vi "MeasurementLink Common Proto Generator.vi"(0 "Proto File Path":path[](array[path]), 1 "Generated Library Full Name":string, 3 "Generate":enum16{"gRPC Server", "gRPC Client", "Both"}(ring), 5 "Import Paths":path[](array[path]), 7 "Prototype Library":path, 9 "Target Project":path, 11 "error in (no error)":errorcluster) -> (15 "error out":errorcluster)   [LabVIEW 2020]
uses:
  <vilib>/regexp/Match Regular Expression.xnode
panel:
  in  "Debug - Prompt before deleting disk content? (F)":bool
  in  "Debug - Leave Project Open? (F)":bool
  # "Ignored for servers as of v0.5.2.2"
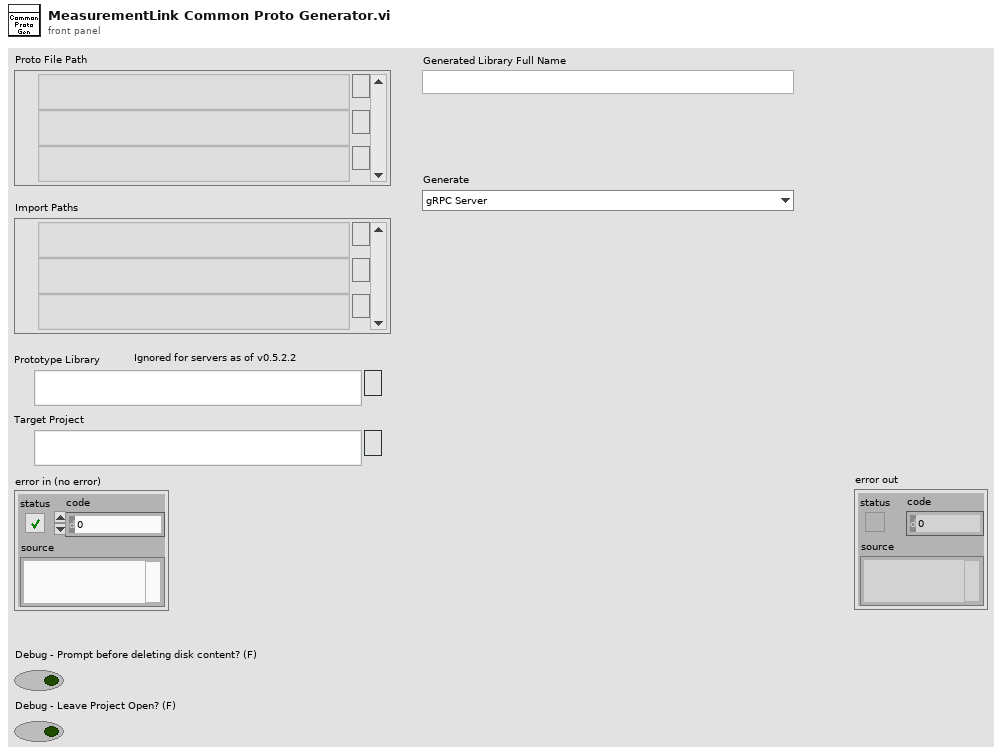
[diagram p1: front panel]
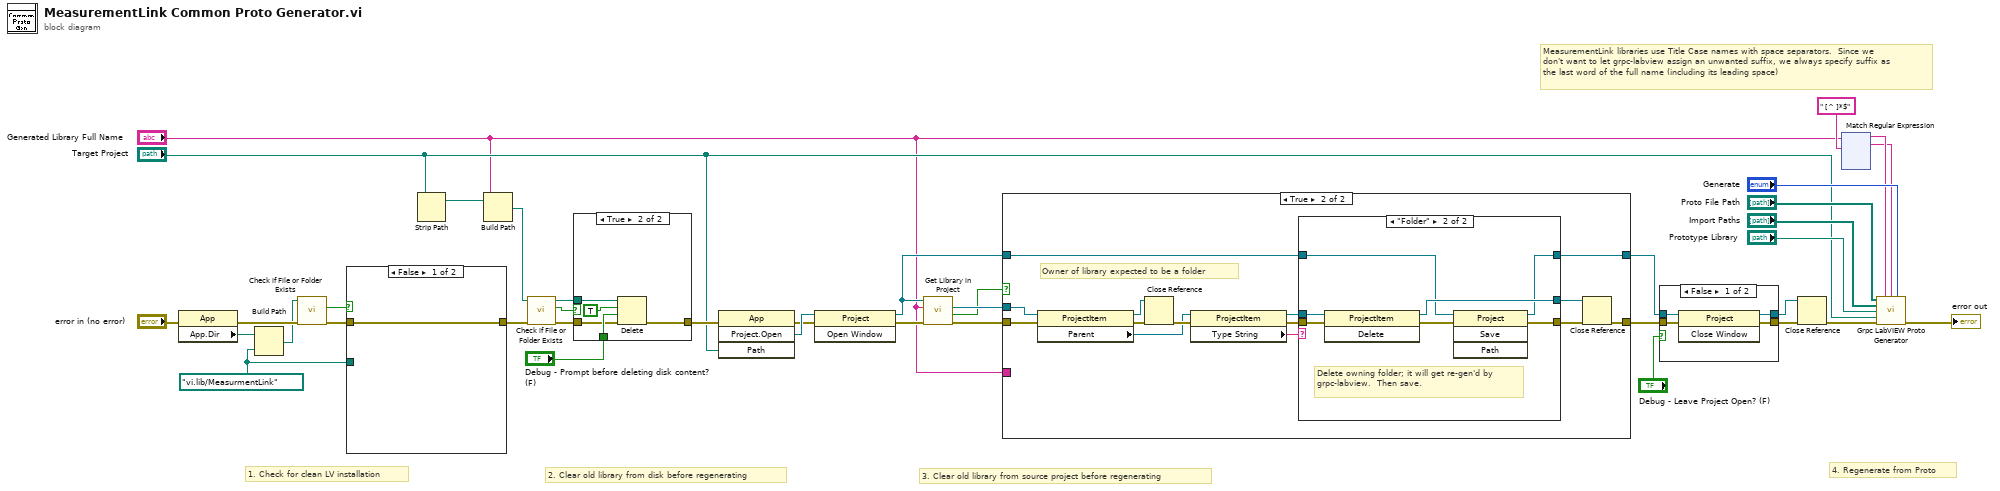
[diagram p0: block diagram]
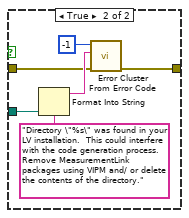
[diagram p2: hidden frame]
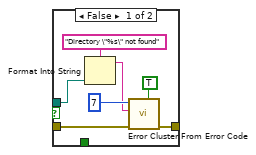
[diagram p3: hidden frame]
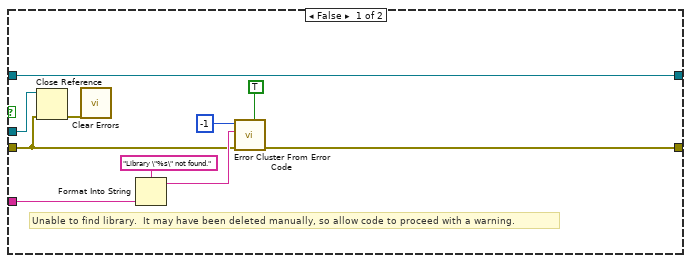
[diagram p4: hidden frame]
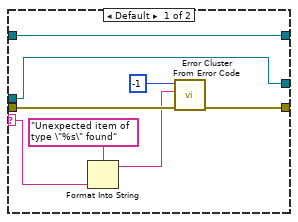
[diagram p5: hidden frame]
diagram:
  w6 = path "vi.lib/MeasurmentLink" ("Target Project")
  # "MeasurementLink libraries use Title Case names with space separators.  Since we don't want to let grpc-labview assign an unwanted suffix, we always specify suffix as the last word of the full name (including its leading space)"
  # "4. Regenerate from Proto"
  # "3. Clear old library from source project before regenerating"
  # "2. Clear old library from disk before regenerating"
  # "1. Check for clean LV installation"
  n1 = property class="App"(error in="error in (no error)") -> (error out=w11:errorcluster, "App.Dir"=w13:path)  [unwired: 1 in, 1 out]
  n2 = Build Path(base path=w13, name or relative path=w6) -> (appended path=w10:path)
  n3 = call <vilib>:"Check if File or Folder Exists.vi"("error in (no error)"=w11, "path"=w10) -> ("error out"=w8:errorcluster, "file or folder exists?"=w9:bool)  [unwired: 7 in, 1 out]
  n4 = case shown="False" w9 {
    tunnel: w8 -> [w39 w42]
    tunnel: [w39 w43] -> w7
    tunnel: w6 -> [_ w40]
    frame False {
    }
    frame True {
      n5 = Format Into String(format string="Directory \"%s\" was found in your LV installation.  This could interfere with the code generation process.  Remove MeasurementLink packages using VIPM and/ or delete the contents of the directory.", w40) -> (resulting string=w44:string)  [unwired: 2 in, 1 out]
      n6 = call <vilib>:"Error Cluster From Error Code.vi"("error in (no error)"=w42, "error message (\"\")"=w44, "error code (0)"=-1) -> ("error out"=w43:errorcluster)  [unwired: 6 in]
    }
  }
  n7 = Strip Path(path="Target Project") -> (stripped path=w15:path)  [unwired: 1 out]
  n8 = Build Path(base path=w15, name or relative path="Generated Library Full Name") -> (appended path=w25:path)
  n9 = call <vilib>:"Check if File or Folder Exists.vi"("error in (no error)"=w7, "path"=w25) -> ("error out"=w24:errorcluster, "file or folder exists?"=w22:bool, "dup path"=w23:path)  [unwired: 7 in]
  n10 = case shown="True" w22 {
    tunnel: [w51 w56] -> w28
    tunnel: "Debug - Prompt before deleting disk content? (F)" -> [_ w55]
    tunnel: w24 -> [w50 w54]
    tunnel: w23 -> [w48 w53]
    frame False {
      n11 = Format Into String(format string="Directory \"%s\" not found", w48) -> (resulting string=w47:string)  [unwired: 2 in, 1 out]
      n12 = call <vilib>:"Error Cluster From Error Code.vi"("is warning? (False)"=TRUE, "error in (no error)"=w50, "error message (\"\")"=w47, "error code (0)"=7) -> ("error out"=w51:errorcluster)  [unwired: 5 in]
    }
    frame True {
      n13 = Delete(path (use dialog)=w53, entire hierarchy (F)=TRUE, confirm (F)=w55, error in=w54) -> (error out=w56:errorcluster)  [unwired: 1 in, 2 out]
    }
  }
  n14 = invoke class="App" method="Project.Open"(error in=w28, "Path"="Target Project") -> (error out=w37:errorcluster, "Project:Open"=w38:refnum<vi>)  [unwired: 2 in, 2 out]
  n15 = invoke class="Project" method="Open Window"(reference=w38, error in=w37) -> (reference out=w29:refnum<vi>, error out=w31:errorcluster)  [unwired: 1 in, 1 out]
  n16 = call "Get Library in Project.vi"("error in (no error)"=w31, "Library Name"="Generated Library Full Name", "Project in"=w29) -> ("error out"=w26:errorcluster, "Found?"=w2:bool, "Measurement Library Item"=w30:refnum<vi>)  [unwired: 6 in]
  n17 = case shown="True" w2 {
    tunnel: w30 -> [w66 w80]
    tunnel: w29 -> [w67 w73]
    tunnel: [w67 w70] -> w36
    tunnel: [w59 w69] -> w35
    tunnel: w26 -> [w60 w68]
    tunnel: "Generated Library Full Name" -> [w58 _]
    frame False {
      # "Unable to find library.  It may have been deleted manually, so allow code to proceed with a warning."
      n18 = Close Reference(reference=w66, error in (no error)=w60) -> (error out=w65:errorcluster)
      n19 = call <vilib>:"Clear Errors.vi"("error in (no error)"=w65) -> ()  [unwired: 5 in, 2 out]
      n20 = Format Into String(format string="Library \"%s\" not found.", w58) -> (resulting string=w62:string)  [unwired: 2 in, 1 out]
      n21 = call <vilib>:"Error Cluster From Error Code.vi"("is warning? (False)"=TRUE, "error in (no error)"=w60, "error message (\"\")"=w62, "error code (0)"=-1) -> ("error out"=w59:errorcluster)  [unwired: 5 in]
    }
    frame True {
      # "Owner of library expected to be a folder"
      n22 = property class="ProjectItem"(reference=w80, error in=w68) -> (reference out=w79:refnum<vi>, error out=w81:errorcluster, "Parent"=w77:refnum<vi>)
      n23 = Close Reference(reference=w79, error in (no error)=w81) -> (error out=w78:errorcluster)
      n24 = property class="ProjectItem"(reference=w77, error in=w78) -> (reference out=w74:refnum<vi>, error out=w75:errorcluster, "Type String"=w76:string)
      n25 = case shown="\"Folder\"" w76 {
        selector: w76 -> [w86 _]
        tunnel: w75 -> [w89 w96]
        tunnel: w74 -> [w83 w95]
        tunnel: [w88 w92] -> w72
        tunnel: w73 -> [w82 w91]
        tunnel: [w82 w90] -> w70
        tunnel: [w83 w94] -> w71
        frame Default {
          n26 = Format Into String(format string="Unexpected item of type \"%s\" found", w86) -> (resulting string=w85:string)  [unwired: 2 in, 1 out]
          n27 = call <vilib>:"Error Cluster From Error Code.vi"("error in (no error)"=w89, "error message (\"\")"=w85, "error code (0)"=-1) -> ("error out"=w88:errorcluster)  [unwired: 6 in]
        }
        frame "Folder" {
          # "Delete owning folder; it will get re-gen'd by grpc-labview.  Then save."
          n28 = invoke class="ProjectItem" method="Delete"(reference=w95, error in=w96) -> (reference out=w94:refnum<vi>, error out=w93:errorcluster)  [unwired: 1 in, 1 out]
          n29 = invoke class="Project" method="Save"(reference=w91, error in=w93) -> (reference out=w90:refnum<vi>, error out=w92:errorcluster)  [unwired: 2 in, 2 out]
        }
      }
      n30 = Close Reference(reference=w71, error in (no error)=w72) -> (error out=w69:errorcluster)
    }
  }
  n31 = case shown="False" "Debug - Leave Project Open? (F)" {
    tunnel: w36 -> [w100 w101]
    tunnel: w35 -> [w99 w102]
    tunnel: [w98 w102] -> w34
    tunnel: [w97 w101] -> w33
    frame False {
      n32 = invoke class="Project" method="Close Window"(reference=w100, error in=w99) -> (reference out=w97:refnum<vi>, error out=w98:errorcluster)  [unwired: 1 in, 1 out]
    }
    frame True {
    }
  }
  n33 = Close Reference(reference=w33, error in (no error)=w34) -> (error out=w21:errorcluster)
  n34 = xnode "Match Regular Expression"("input string"="Generated Library Full Name", "regular expression"=" [^ ]*$") -> ("before match"=w4:string, "whole match"=w3:string)  [unwired: 4 in, 3 out]
  n35 = call "Grpc LabVIEW Proto Generator.vi"("Proto File Path"="Proto File Path", "Generated Library Name"=w4, "Library Suffix"=w3, "Generate"="Generate", "Import Paths"="Import Paths", "Prototype Library"="Prototype Library", "Target Project"="Target Project", "error in (no error)"=w21) -> ("error out"=→"error out":errorcluster)  [unwired: 7 in]
